vi "Numeric_Create.vi"(0 "reference in":refnum<class "Numeric.lvclass">, 1 "Object Attributes":T2, 2 "Control Attributes":T4, 3 "Graph Attributes":T1, 5 "error in (no error)":errorcluster) -> (14 "reference out":refnum<class "Numeric.lvclass">, 19 "error out":errorcluster)   [LabVIEW 2014, in "Numeric.lvclass"]
uses:
  Numeric.lvclass
  Control_class/Attributes.ctl
  Text_class/Text.lvclass
  Object_class/Attributes.ctl
  Object_class/Coordinates.ctl
  Attributes.ctl
  Control_class/Control.lvclass
  Object_class/Object.lvclass
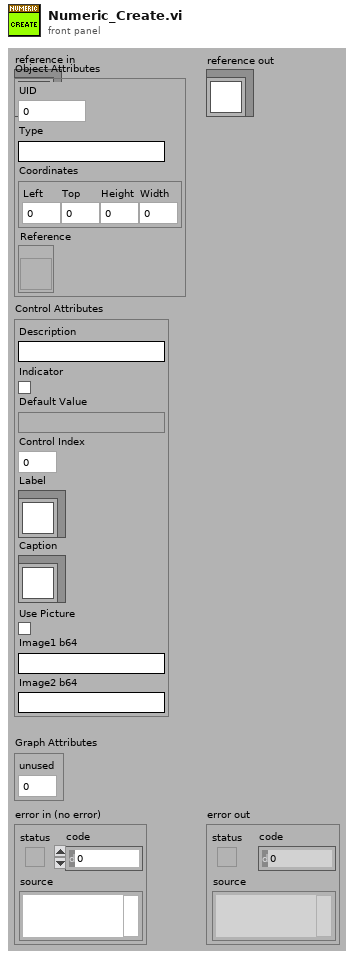
[diagram p1: front panel]
types:
  T1 = typedef "Numeric.lvclass/Attributes.ctl" = cluster{"unused":dbl}
  T2 = typedef "Object.lvclass/Attributes.ctl" = cluster{"UID":i32, "Type":string, "Coordinates":T3, "Reference":refnum<vi>}
  T3 = typedef "Object.lvclass/Coordinates.ctl" = cluster{"Left":i32, "Top":i32, "Height":u32, "Width":u32}
  T4 = typedef "Control.lvclass/Attributes.ctl" = cluster{"Description":string, "Indicator":bool, "Default Value":variant, "Control Index":i32, "Label":refnum<class "Text.lvclass">, "Caption":refnum<class "Text.lvclass">, "Use Picture":bool, "Image1 b64":string, "Image2 b64":string}
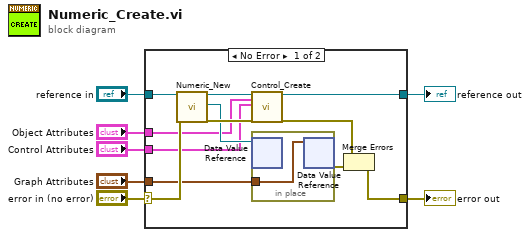
[diagram p0: block diagram]
diagram:
  n1 = case shown="No Error" "error in (no error)" {
    selector: "error in (no error)" -> [w18 w22]
    tunnel: [w16 w22] -> w6
    tunnel: "reference in" -> [w19 w21]
    tunnel: [w13 w21] -> w4
    tunnel: "Object Attributes" -> [w11 _]
    tunnel: "Control Attributes" -> [w9 _]
    tunnel: "Graph Attributes" -> [w8 _]
    frame No Error {
      n2 = call "Numeric_New.vi"("reference in"=w19, "error in (no error)"=w18) -> ("reference out"=w15:refnum<class "Numeric.lvclass">, "DVRRefOut"=w12:refnum<data-value>, "error out"=w14:errorcluster)  [unwired: 14 in, 1 out]
      n3 = call "Control_Create.vi"("reference in"=w15, "Object Attributes"=w11, "Control Attributes"=w9, "error in (no error)"=w14) -> ("reference out"=w13:refnum<class "Numeric.lvclass">, "error out"=w10:errorcluster)  [unwired: 14 in]
      n4 = in-place {
        in-place-border: w8 -> [w20]
        n5 = in-place-dvr #1(w12) -> ()  [unwired: 2 out]
        n6 = in-place-dvr #1(w20) -> (w17:errorcluster)  [unwired: 1 out]
      }
      n7 = Merge Errors(w10, w17) -> (w16:errorcluster)
    }
    frame Error {
    }
  }
  "error out" <- w6
  "reference out" <- w4
